vi "database_connection_write_dev_MQTT_database_array_V2.vi"(6 "connection reference":T2, 7 "string":string="Raw.DMG_MORI_DMU_40_EVO", 8 "error in (no error)":errorcluster, 9 "data 2":dbl[](array[numeric]), 10 "Machine Data":T3={"Zload"="", "Yload"="", "Xload"="", "path_position"="", "Fovr"="", "SspeedOvr"="", "Program Name"="", "Program status"="", "Block of code being executed"="", "Line of code"="", "Machine availability"="", "Emergency status"="", "Controller mode"="", "Tool_id"="UNAVAILABLE"}, 11 "current time 2":timestamp format="%^<%Y-%m-%d %H:%M:%S%3u>T") -> (0 "connection reference out":T2, 3 "error out":errorcluster)   [LabVIEW 2017]
uses:
  <vilib>/addons/database/Connection.llb/Conn ObjectReference.ctl
  data_base_structure_V2.ctl
  data_base_structure.ctl
  controls/databse_structure.ctl
  <vilib>/addons/database/NI_Database_API.lvlib
panel:
  out "output cluster":T1
  out "Array":string[](array[string])=["timestamp", "available", "execution", "controller_mode", "spindle_load", "spindle_speed", "sspeedovr", "feed_rate", "fovr", "I_part", "J_part", "K_part", "Xpos_part", "Ypos_part", "Zpos_part", "Apos_machine", "Bpos_machine", "Xload", "Yload", "Zload", "Aload", "Bload", "tool_id", "program_number", "program_name", "block_code", "line_number", "estop", "accel_x_rms", "accel_y_rms", "accel_z_rms"]
  out "Program Name":string
  out "date/time string 2":string
  out "ISO-8601 UTC Formatted DateTime String":string
  out "error out 2":errorcluster
  in  "error in":errorcluster
  out "Timestamp":timestamp
  out "date/time string":string
  out "current time 3":timestamp
  out "resulting string 2":string
  out "Xload":string
  out "Machine availability":string
  out "resulting string":string
  out "output array 2":dbl[](array[numeric])
  out "size(s) 2":i32
  out "valueSent 2":string="14:19:17.238_"
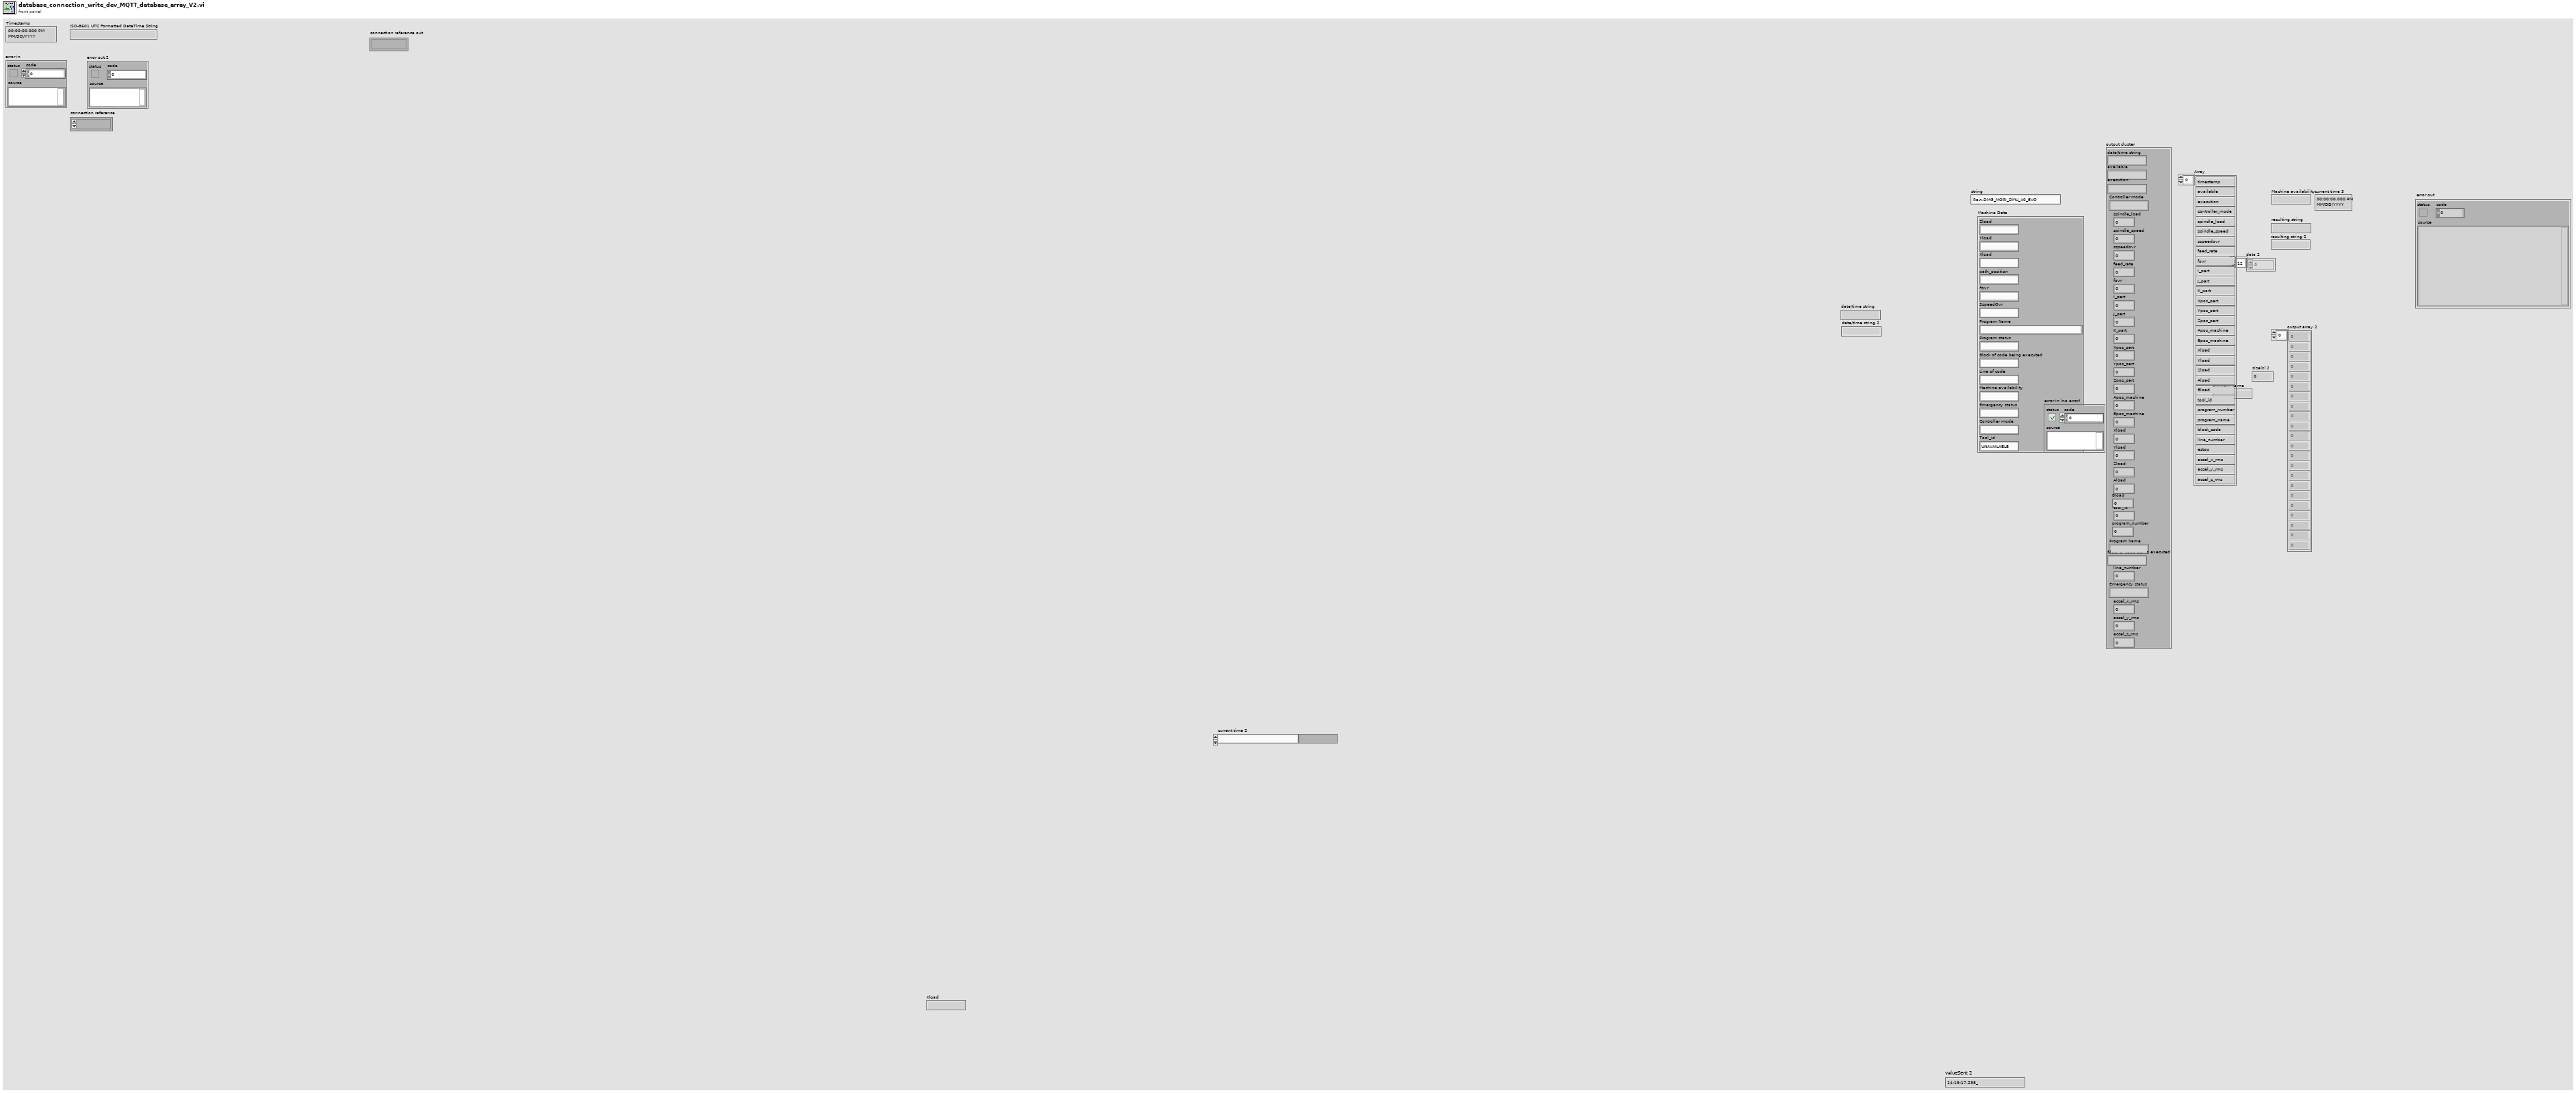
[diagram p1: front panel]
types:
  T1 = typedef "data_base_structure_V2.ctl" = cluster{"date/time string":string, "available":string, "Controller mode":string, "spindle_load":dbl, "spindle_speed":dbl, "sspeedovr":dbl, "feed_rate":dbl, "fovr":dbl, "I_part":dbl, "J_part":dbl, "K_part":dbl, "Xpos_part":dbl, "Ypos_part":dbl, "Zpos_part":dbl, "Apos_machine":dbl, "Bpos_machine":dbl, "Xload":dbl, "Yload":dbl, "Zload":dbl, "Aload":dbl, "Bload":dbl, "tool_id":dbl, "program_number":dbl, "Program Name":string, "Block of code being executed":string, "line_number":dbl, "Emergency status":string, "accel_x_rms":dbl, "accel_y_rms":dbl, "accel_z_rms":dbl, "execution":string}
  T2 = typedef "NI_Database_API.lvlib/Conn ObjectReference.ctl" = refnum<k1>
  T3 = cluster{"Zload":string, "Yload":string, "Xload":string, "path_position":string, "Fovr":string, "SspeedOvr":string, "Program Name":string, "Program status":string, "Block of code being executed":string, "Line of code":string, "Machine availability":string, "Emergency status":string, "Controller mode":string, "Tool_id":string}
  T4 = typedef "data_base_structure.ctl" = cluster{"available ":dbl, "controller_mode":string, "spindle_load":dbl, "spindle_speed ":dbl, "sspeedovr":dbl, "J_part":dbl, "K_part":dbl, "Xpos_part":dbl, "Ypos_part":dbl, "Zpos_part":dbl, "Apos_machine":dbl, "Bpos_machine":dbl, "Xload":dbl, "Yload":dbl, "Zload":dbl, "Aload":dbl, "Bload":dbl, "tool_id":dbl, "program_name":string, "block_code":string, "line_number":dbl, "estop":string, "accel_x_rms":dbl, "accel_y_rms":dbl, "accel_z_rms":dbl, "program_number":dbl, "timestamp":string, "feed_rate ":dbl, "fovr":dbl, "I_part ":dbl}
  T5 = cluster{"date/time string":string, "available":string, "execution":string, "Controller mode":string, "spindle_load":dbl, "spindle_speed":dbl, "sspeedovr":dbl, "feed_rate":dbl, "fovr":dbl, "I_part":dbl, "J_part":dbl, "K_part":dbl, "Xpos_part":dbl, "Ypos_part":dbl, "Zpos_part":dbl, "Apos_machine":dbl, "Bpos_machine":dbl, "Xload":dbl, "Yload":dbl, "Zload":dbl, "Aload":dbl, "Bload":dbl, "tool_id":dbl, "program_number":dbl, "Program Name":string, "Block of code being executed":string, "line_number":dbl, "Emergency status":string, "accel_x_rms":dbl, "accel_y_rms":dbl, "accel_z_rms":dbl}
  T6 = typedef "databse_structure.ctl" = cluster{"date/time string":string, "available":string, "execution":string, "Controller mode":string, "accel_z_rms":dbl, "accel_y_rms":dbl, "accel_x_rms":dbl, "Emergency status":string, "line_number":dbl, "Block of code being executed":string, "Program Name":string, "program_number":dbl, "tool_id":dbl, "Bload":dbl, "Aload":dbl, "Zload":dbl, "Yload":dbl, "Xload":dbl, "Bpos_machine":dbl, "Apos_machine":dbl, "Zpos_part":dbl, "Ypos_part":dbl, "Xpos_part":dbl, "K_part":dbl, "J_part":dbl, "I_part":dbl, "fovr":dbl, "feed_rate":dbl, "sspeedovr":dbl, "spindle_speed":dbl, "spindle_load":dbl}
  T7 = cluster{"data 2[0]":dbl, "data 2[1]":dbl, "data 2[2]":dbl, "data 2[3]":dbl, "data 2[4]":dbl, "data 2[5]":dbl, "data 2[6]":dbl, "data 2[7]":dbl, "data 2[8]":dbl, "data 2[9]":dbl, "data 2[10]":dbl, "data 2[11]":dbl, "data 2[12]":dbl, "data 2[13]":dbl, "data 2[14]":dbl, "data 2[15]":dbl, "data 2[16]":dbl, "data 2[17]":dbl, "data 2[18]":dbl, "data 2[19]":dbl, "data 2[20]":dbl, "data 2[21]":dbl}
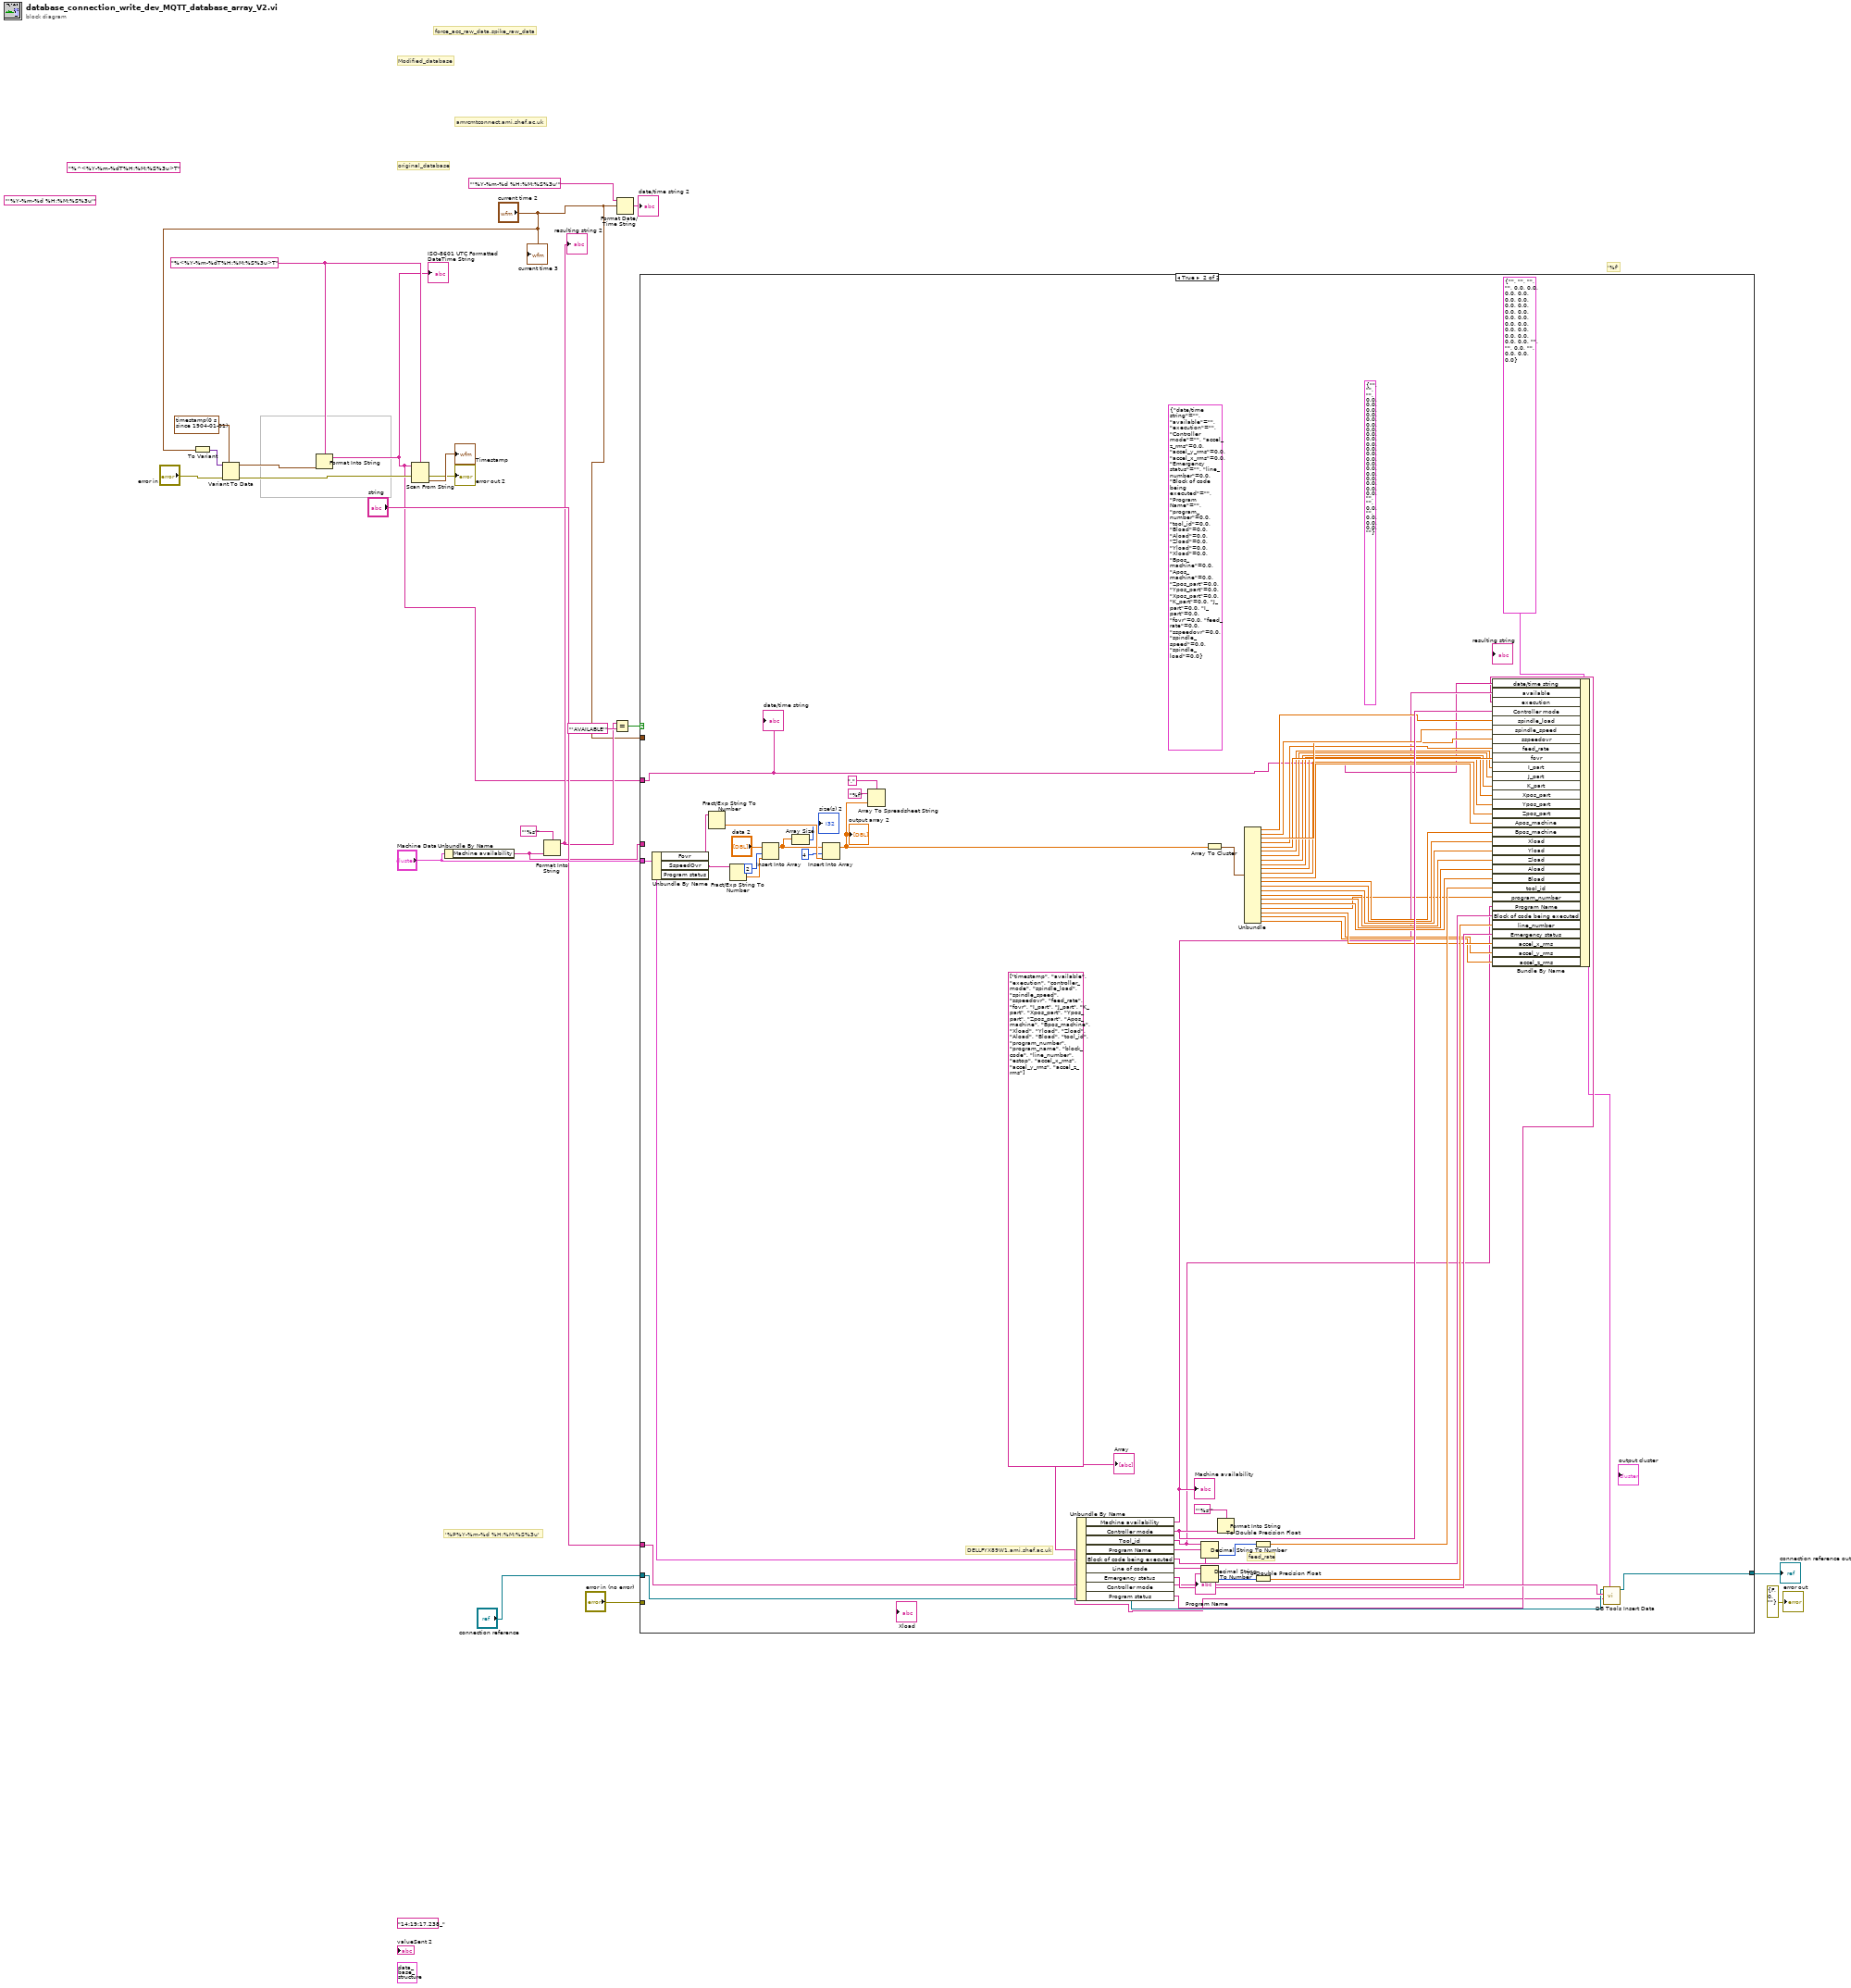
[diagram p0: block diagram]
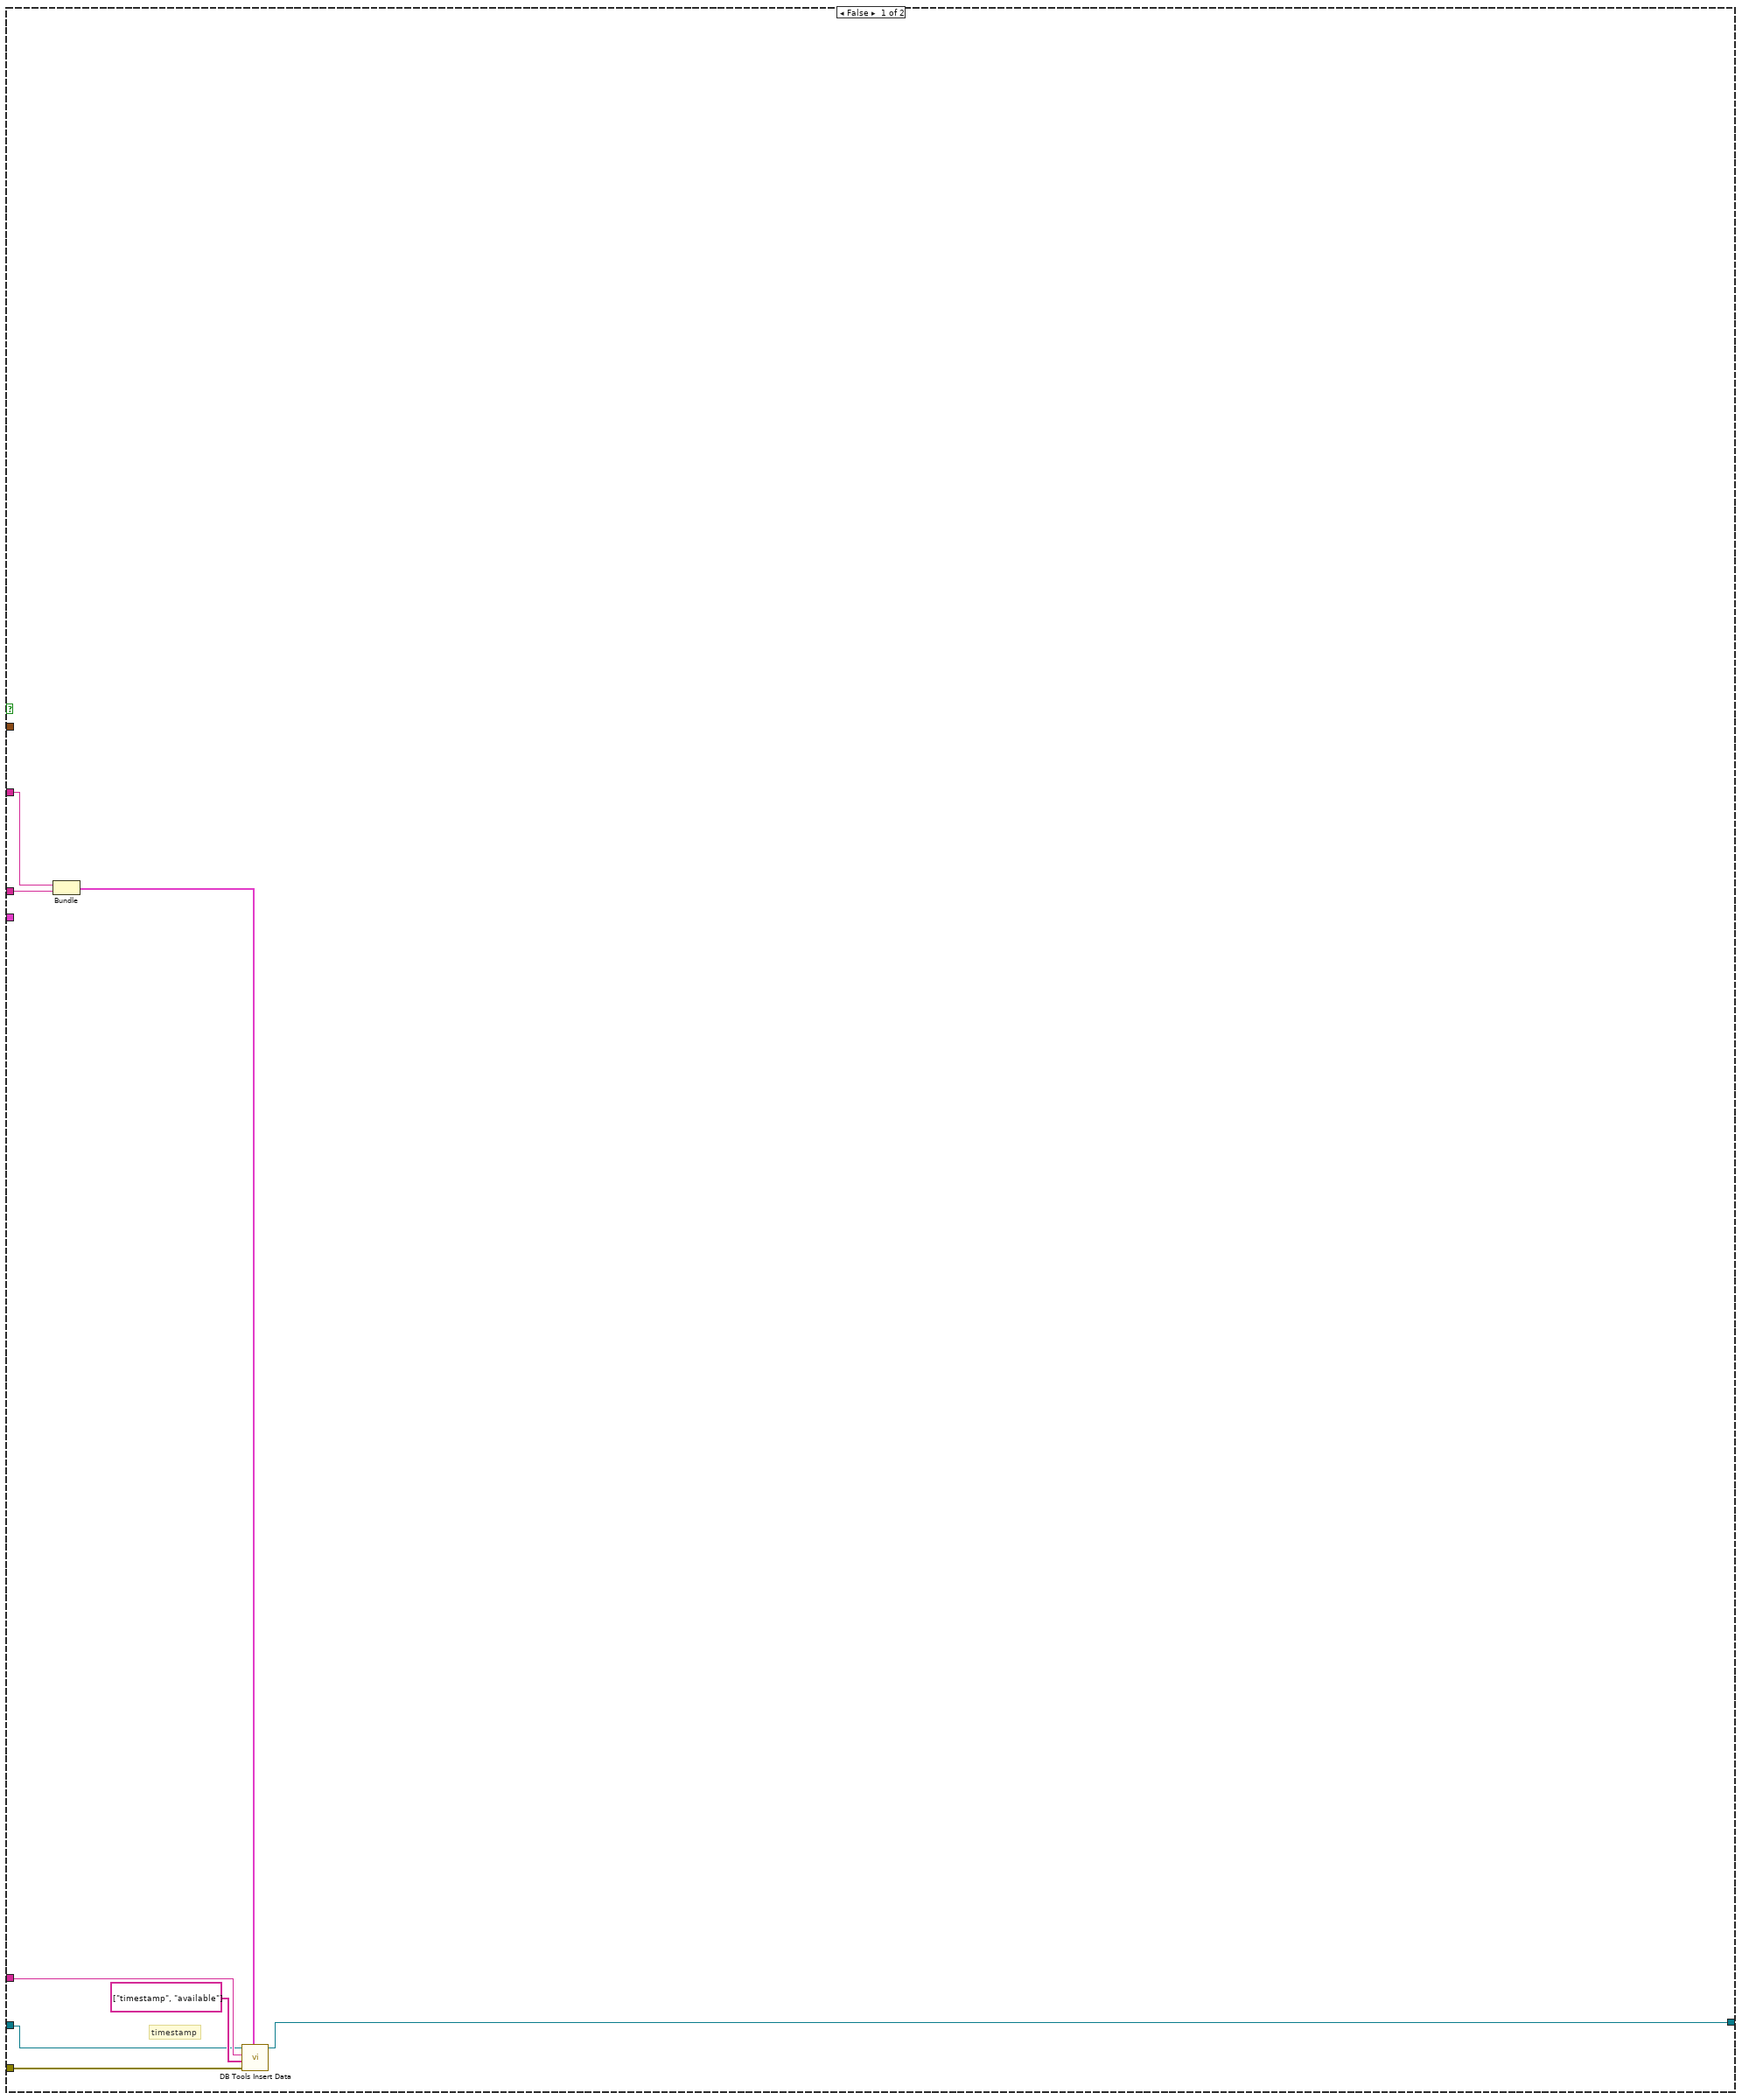
[diagram p2: hidden frame]
diagram:
  (unwired) "%^<%Y-%m-%dT%H:%M:%S%3u>T" ("format string")
  (unwired) "'%Y-%m-%d %H:%M:%S%3u'" ("time format string (%c)")
  w9 = "%<%Y-%m-%dT%H:%M:%S%3u>T" ("format string")
  (unwired) "14:19:17.238_" ("valueSent 2")
  (unwired) T4 {"available "=0.0, "controller_mode"="", "spindle_load"=0.0, "spindle_speed "=0.0, "sspeedovr"=0.0, "J_part"=0.0, "K_part"=0.0, "Xpos_part"=0.0, "Ypos_part"=0.0, "Zpos_part"=0.0, "Apos_machine"=0.0, "Bpos_machine"=0.0, "Xload"=0.0, "Yload"=0.0, "Zload"=0.0, "Aload"=0.0, "Bload"=0.0, "tool_id"=0.0, "program_name"="", "block_code"="", "line_number"=0.0, "estop"="", "accel_x_rms"=0.0, "accel_y_rms"=0.0, "accel_z_rms"=0.0, "program_number"=0.0, "timestamp"="", "feed_rate "=0.0, "fovr"=0.0, "I_part "=0.0} ("Cluster")
  # "'%P%Y-%m-%d %H:%M:%S%3u'"
  # "'%f'"
  # "original_database"
  # "force_acc_raw_data,spike_raw_data"
  # "Modified_database"
  # "amrcmtconnect.ami.shef.ac.uk"
  n1 = To Variant(anything="current time 2") -> (Variant=w14:variant)
  n2 = Variant To Data(error in="error in", type=timestamp(0 s since 1904-01-01) ("time stamp"), Variant=w14) -> (data=w8:timestamp, error out=w11:errorcluster)
  n3 = Format Into String(format string=w9, w8) -> (resulting string=w6:string)  [unwired: 2 in, 1 out]
  "ISO-8601 UTC Formatted DateTime String" <- w6
  n4 = Scan From String(format string=w9, input string=w6, error in=w11) -> (error out=→"error out 2":errorcluster, output 1=→"Timestamp":timestamp)  [unwired: 2 in, 2 out]
  n5 = Unbundle By Name("Machine Data") -> ("Machine availability"=w2:string)
  n6 = Format Into String(format string="'%s'", w2) -> (resulting string=w16:string)  [unwired: 2 in, 1 out]
  "resulting string 2" <- w16
  n7 = Equal?(x=w16, y="'AVAILABLE'") -> (x = y?=w19:bool)
  n8 = Format Date/Time String(time format string (%c)="'%Y-%m-%d %H:%M:%S%3u'", seconds (now)="current time 2") -> (date/time string=→"date/time string 2":string)  [unwired: 1 in]
  n9 = case shown="True" w19 {
    tunnel: "Machine Data" -> [_ w43]
    tunnel: "error in (no error)" -> [w26 _]
    tunnel: "string" -> [w31 w42]
    tunnel: w2 -> [w24 _]
    tunnel: "current time 2" -> [_ _]
    tunnel: w6 -> [w28 w41]
    tunnel: "connection reference" -> [w27 w40]
    tunnel: [w25 w39] -> w3
    frame False {
      # "timestamp"
      n10 = Bundle(w28, "Machine availability"=w24) -> (w29:cluster{string, "Machine availability":string})  [unwired: 1 in]
      n11 = call <vilib>:"DB Tools Insert Data.vi"("data"=w29, "error in (no error)"=w26, "columns"=string[] ["timestamp", "available"], "table"=w31, "connection reference"=w27) -> ("connection reference out"=w25:T2)  [unwired: 5 in, 1 out]
    }
    frame True {
      (unwired) T6 {"date/time string"="", "available"="", "execution"="", "Controller mode"="", "accel_z_rms"=0.0, "accel_y_rms"=0.0, "accel_x_rms"=0.0, "Emergency status"="", "line_number"=0.0, "Block of code being executed"="", "Program Name"="", "program_number"=0.0, "tool_id"=0.0, "Bload"=0.0, "Aload"=0.0, "Zload"=0.0, "Yload"=0.0, "Xload"=0.0, "Bpos_machine"=0.0, "Apos_machine"=0.0, "Zpos_part"=0.0, "Ypos_part"=0.0, "Xpos_part"=0.0, "K_part"=0.0, "J_part"=0.0, "I_part"=0.0, "fovr"=0.0, "feed_rate"=0.0, "sspeedovr"=0.0, "spindle_speed"=0.0, "spindle_load"=0.0}
      w34 = string[] ["timestamp", "available", "execution", "controller_mode", "spindle_load", "spindle_speed", "sspeedovr", "feed_rate", "fovr", "I_part", "J_part", "K_part", "Xpos_part", "Ypos_part", "Zpos_part", "Apos_machine", "Bpos_machine", "Xload", "Yload", "Zload", "Aload", "Bload", "tool_id", "program_number", "program_name", "block_code", "line_number", "estop", "accel_x_rms", "accel_y_rms", "accel_z_rms"]
      (unwired) T1 {"date/time string"="", "available"="", "Controller mode"="", "spindle_load"=0.0, "spindle_speed"=0.0, "sspeedovr"=0.0, "feed_rate"=0.0, "fovr"=0.0, "I_part"=0.0, "J_part"=0.0, "K_part"=0.0, "Xpos_part"=0.0, "Ypos_part"=0.0, "Zpos_part"=0.0, "Apos_machine"=0.0, "Bpos_machine"=0.0, "Xload"=0.0, "Yload"=0.0, "Zload"=0.0, "Aload"=0.0, "Bload"=0.0, "tool_id"=0.0, "program_number"=0.0, "Program Name"="", "Block of code being executed"="", "line_number"=0.0, "Emergency status"="", "accel_x_rms"=0.0, "accel_y_rms"=0.0, "accel_z_rms"=0.0, "execution"=""} ("cluster")
      # "feed_rate"
      # "DELLFYX89W1.ami.shef.ac.uk"
      n12 = Unbundle By Name(w43) -> ("Fovr"=w79:string, "SspeedOvr"=w84:string)  [unwired: 1 out]
      n13 = Fract/Exp String To Number(string=w79) -> (number=w81:dbl)  [unwired: 3 in, 1 out]
      n14 = Fract/Exp String To Number(string=w84) -> (number=w83:dbl)  [unwired: 3 in, 1 out]
      n15 = Insert Into Array(array="data 2", index=2, new element=w83) -> (w77:dbl[])
      n16 = Array Size(array=w77) -> (size(s)=→"size(s) 2":i32)
      n17 = Insert Into Array(array=w77, index=4, new element=w81) -> (w72:dbl[])
      "output array 2" <- w72
      n18 = Array To Spreadsheet String(delimiter (Tab)=",", array=w72, 3:"%f" ("format string")) -> ()  [unwired: 1 out]
      n19 = Unbundle By Name(w43) -> ("Machine availability"=w44:string, "Controller mode"=w70:string, "Tool_id"=w36:string, "Program Name"=→"Program Name":string, "Block of code being executed"=w50:string, "Line of code"=w75:string, "Emergency status"=w48:string, "Program status"=w35:string)  [unwired: 1 out]
      "Machine availability" <- w44
      n20 = Decimal String To Number(string=w36) -> (number=w76:i32)  [unwired: 2 in, 1 out]
      n21 = Decimal String To Number(string=w75) -> (number=w74:i32)  [unwired: 2 in, 1 out]
      n22 = Array To Cluster(array=w72) -> (cluster=w71:T7)
      n23 = Format Into String(format string="'%s'", w70) -> ()  [unwired: 2 in, 2 out]
      n24 = Unbundle(w71) -> ("data 2[0]"=w69:dbl, "data 2[1]"=w68:dbl, "data 2[2]"=w67:dbl, "data 2[3]"=w66:dbl, "data 2[4]"=w65:dbl, "data 2[5]"=w64:dbl, "data 2[6]"=w63:dbl, "data 2[7]"=w62:dbl, "data 2[8]"=w61:dbl, "data 2[9]"=w60:dbl, "data 2[10]"=w59:dbl, "data 2[11]"=w58:dbl, "data 2[12]"=w57:dbl, "data 2[13]"=w56:dbl, "data 2[14]"=w55:dbl, "data 2[15]"=w54:dbl, "data 2[16]"=w53:dbl, "data 2[17]"=w52:dbl, "data 2[18]"=w37:dbl, "data 2[19]"=w47:dbl, "data 2[20]"=w46:dbl, "data 2[21]"=w45:dbl)
      n25 = To Double Precision Float(number=w76) -> (double precision float=w51:dbl)
      n26 = To Double Precision Float(number=w74) -> (double precision float=w49:dbl)
      n27 = Bundle By Name(cluster=T5 {"date/time string"="", "available"="", "execution"="", "Controller mode"="", "spindle_load"=0.0, "spindle_speed"=0.0, "sspeedovr"=0.0, "feed_rate"=0.0, "fovr"=0.0, "I_part"=0.0, "J_part"=0.0, "K_part"=0.0, "Xpos_part"=0.0, "Ypos_part"=0.0, "Zpos_part"=0.0, "Apos_machine"=0.0, "Bpos_machine"=0.0, "Xload"=0.0, "Yload"=0.0, "Zload"=0.0, "Aload"=0.0, "Bload"=0.0, "tool_id"=0.0, "program_number"=0.0, "Program Name"="", "Block of code being executed"="", "line_number"=0.0, "Emergency status"="", "accel_x_rms"=0.0, "accel_y_rms"=0.0, "accel_z_rms"=0.0}, "date/time string"=w41, "available"=w44, "execution"=w35, "Controller mode"=w70, "spindle_load"=w69, "spindle_speed"=w68, "sspeedovr"=w67, "feed_rate"=w66, "fovr"=w65, "I_part"=w64, "J_part"=w63, "K_part"=w62, "Xpos_part"=w61, "Ypos_part"=w60, "Zpos_part"=w59, "Apos_machine"=w58, "Bpos_machine"=w57, "Xload"=w56, "Yload"=w55, "Zload"=w54, "Aload"=w53, "Bload"=w52, "tool_id"=w51, "program_number"=w37, "Program Name"=w36, "Block of code being executed"=w50, "line_number"=w49, "Emergency status"=w48, "accel_x_rms"=w47, "accel_y_rms"=w46, "accel_z_rms"=w45) -> (w33:T5)
      n28 = call <vilib>:"DB Tools Insert Data.vi"("data"=w33, "columns"=w34, "table"=w42, "connection reference"=w40) -> ("connection reference out"=w39:T2)  [unwired: 6 in, 1 out]
      "date/time string" <- w41
      "Array" <- w34
    }
  }
  "connection reference out" <- w3
  "error out" <- errorcluster {"status"=FALSE, "code"=0, "source"=""} ("error out")
  "current time 3" <- "current time 2"
